vi "fpga_LP1ControlUnit (P Class).vi"(0 "#Ch":fxp<+,5,5>, 1 "reset":bool, 2 "input valid":bool) -> (5 "ready for input":bool, 6 "procInputValid":bool, 7 "output valid":bool, 8 "opState":T1, 9 "coefRDAddr":fxp<+,6,6>)   [LabVIEW 2013, in "NI_EP_PMU_FPGA.lvlib"]
uses:
  <vilib>/addons/Electrical Power/PMU/NI_EP_PMU_FPGA.lvlib
  <vilib>/rvi/FXPMathLib/basic elements/FxpDiscreteDelay/XNode/nifxpmath_DiscreteDelay.xnode
  <vilib>/rvi/FXPMathLib/basic elements/FxpAddSub/XNode/nifxpmath_AddSub.xnode
  <vilib>/rvi/FXPMathLib/sim/FxpSim.dll
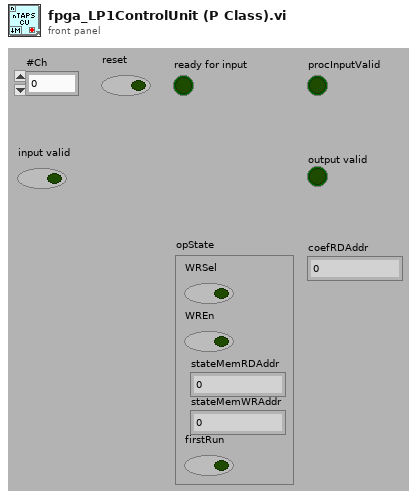
[diagram p1: front panel]
types:
  T1 = cluster{"WRSel":bool, "WREn":bool, "stateMemRDAddr":fxp<+,8,8>, "stateMemWRAddr":fxp<+,8,8>, "firstRun":bool}
  T2 = cluster{"idle":bool, "ready for input":bool, "macCnt":fxp<+,4,4>, "chCnt":fxp<+,5,5>, "phaseCnt":fxp<+,4,4>, "WRPageAddr":fxp<+,8,8>, "WRBaseAddr":fxp<+,8,8>, "first run?":bool}
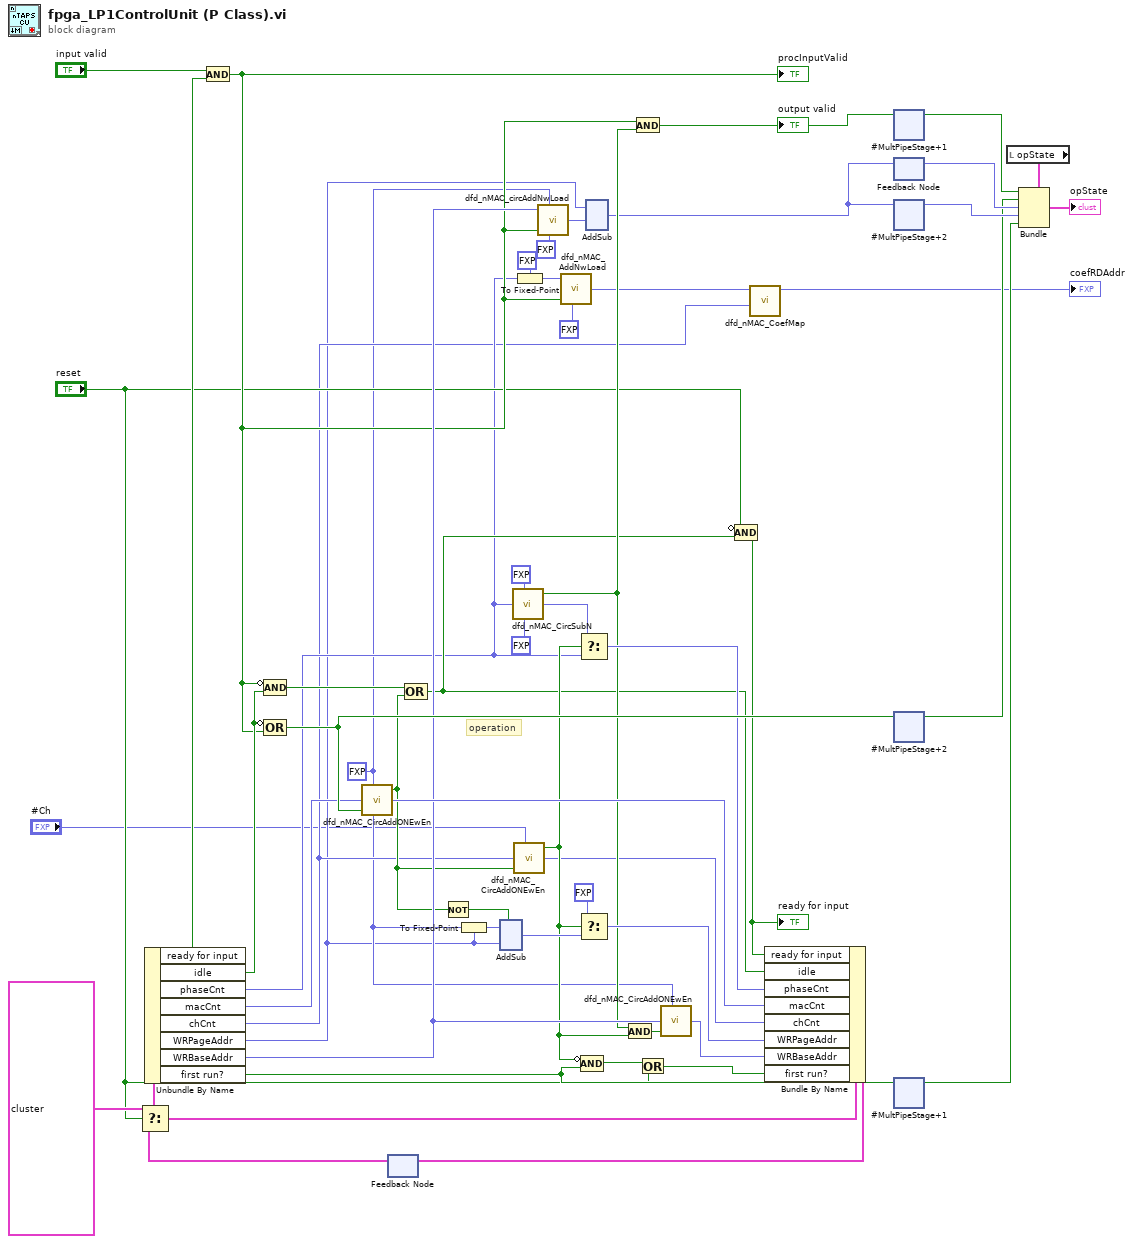
[diagram p0: block diagram]
diagram:
  w4 = fxp<+,4,4> 8.0 ("#TPPM")
  # "operation"
  n1 = feedback #1() -> (w40:T2)  [unwired: 1 out]
  n2 = Select(t=T2 {"idle"=TRUE, "ready for input"=FALSE, "macCnt"=0.0, "chCnt"=0.0, "phaseCnt"=0.0, "WRPageAddr"=0.0, "WRBaseAddr"=0.0, "first run?"=TRUE} ("CUInitialState"), s="reset", f=w40) -> (s? t:f=w42:T2)
  n3 = Unbundle By Name(w42) -> ("ready for input"=w24:bool, "idle"=w31:bool, "phaseCnt"=w11:fxp<+,4,4>, "macCnt"=w38:fxp<+,4,4>, "chCnt"=w5:fxp<+,5,5>, "WRPageAddr"=w2:fxp<+,8,8>, "WRBaseAddr"=w35:fxp<+,8,8>, "first run?"=w19:bool)
  n4 = And(x="input valid", y=w24) -> (x .and. y?=w23:bool)
  "procInputValid" <- w23
  n5 = Compound Arithmetic op=AND(invert w23, w31) -> (w48:bool)
  n6 = Compound Arithmetic op=OR(invert w31, w23) -> (w45:bool)
  n7 = call "dfd_nMAC_CircAddONEwEn.vi"("len"=w4, "idxIn"=w38, "Enable"=w45) -> ("wrap?"=w20:bool, "idxOut"=w37:fxp<+,4,4>)  [unwired: 5 in]
  n8 = Compound Arithmetic op=OR(w48, w20) -> (w21:bool)
  n9 = Not(x=w20) -> (.not. x?=w53:bool)
  n10 = To Fixed-Point ("ToCoef")(fixed-point type=w2, number=w4) -> (fixed-point=w3:fxp<+,8,8>)
  n11 = xnode ("AddSub")("x"=w3, "y"=w2, "use zero instead of x"=w53) -> ("s"=w51:fxp<+,8,8>)  [unwired: 1 out]
  n12 = call "dfd_nMAC_CircSubN.vi"("len"=fxp<+,4,4> 8.0 ("#M"), "idxIn"=w11, "step"=fxp<+,1,1> 1.0 ("#L")) -> ("wrap?"=w33:bool, "idxOut"=w32:fxp<+,4,4>)  [unwired: 5 in]
  n13 = call "dfd_nMAC_CircAddONEwEn.vi"("len"="#Ch", "idxIn"=w5, "Enable"=w20) -> ("wrap?"=w29:bool, "idxOut"=w22:fxp<+,5,5>)  [unwired: 5 in]
  n14 = To Fixed-Point ("ToCoef")(fixed-point type=fxp<+,6,6> 0.0 ("CoefAddr"), number=w11) -> (fixed-point=w13:fxp<+,6,6>)
  n15 = call "dfd_nMAC_circAddNwLoad.vi"("initIdx"=w35, "len"=w4, "load"=w23, "step"=fxp<+,1,1> 1.0) -> ("idxOut"=w15:fxp<+,8,8>)  [unwired: 5 in]
  n16 = call "dfd_nMAC_AddNwLoad.vi"("initIdx"=w13, "load"=w23, "step"=fxp<+,4,4> 8.0 ("#M")) -> ("idxOut"=w7:fxp<+,6,6>)  [unwired: 6 in]
  n17 = Select(t=w32, s=w29, f=w11) -> (s? t:f=w39:fxp<+,4,4>)
  n18 = Select(t=fxp<+,1,1> 0.0, s=w29, f=w51) -> (s? t:f=w36:fxp<+,8,8>)
  n19 = Compound Arithmetic op=AND(invert w29, w19) -> (w27:bool)
  n20 = xnode ("AddSub")("x"=w2, "y"=w15) -> ("s"=w14:fxp<+,8,8>)  [unwired: 1 out]
  n21 = And(x=w33, y=w29) -> (x .and. y?=w50:bool)
  n22 = And(x=w23, y=w33) -> (x .and. y?=w26:bool)
  "output valid" <- w26
  n23 = Or(x=w27, y="reset") -> (x .or. y?=w28:bool)
  n24 = call "dfd_nMAC_CircAddONEwEn.vi"("len"=w4, "idxIn"=w35, "Enable"=w50) -> ("idxOut"=w34:fxp<+,8,8>)  [unwired: 5 in, 1 out]
  n25 = Compound Arithmetic op=AND(invert "reset", w21) -> (w17:bool)
  "ready for input" <- w17
  n26 = call "dfd_nMAC_CoefMap.vi"("chCnt"=w5, "coefOffsetAddr"=w7) -> ("coefRDAddr"=→"coefRDAddr":fxp<+,6,6>)  [unwired: 9 in]
  n27 = Bundle By Name(cluster=w42, "ready for input"=w17, "idle"=w21, "phaseCnt"=w39, "macCnt"=w37, "chCnt"=w22, "WRPageAddr"=w36, "WRBaseAddr"=w34, "first run?"=w28) -> (w41:T2)
  n28 = feedback-in #1(w41) -> ()
  n29 = xnode ("#MultPipeStage+1")("D"=w26) -> ("Q"=w25:bool)
  n30 = feedback-in #2(w14) -> ()
  n31 = feedback #2() -> (w47:fxp<+,8,8>)  [unwired: 1 out]
  n32 = xnode ("#MultPipeStage+2")("D"=w14) -> ("Q"=w46:fxp<+,8,8>)
  n33 = xnode ("#MultPipeStage+2")("D"=w45) -> ("Q"=w44:bool)
  n34 = xnode ("#MultPipeStage+1")("D"=w19) -> ("Q"=w8:bool)
  n35 = local read "opState"() -> (w10:T1)
  n36 = Bundle(cluster=w10, "WRSel"=w25, "WREn"=w44, "stateMemRDAddr"=w47, "stateMemWRAddr"=w46, "firstRun"=w8) -> (→"opState":T1)
